vi "SwerveModuleOdometry.vi"(4 "Robot Heading(deg)":dbl, 6 "Wheel Distance (m)":dbl, 7 "Wheel Azimuth (deg)":dbl, 9 "Velocity (m/s)":dbl) -> (0 "Delta Y (m)":dbl, 1 "Delta X (m)":dbl, 2 "Velocity Y (m/s)":dbl, 3 "Velocity X (m/s)":dbl)   [LabVIEW 2020]
doc: "This VI calculates the odometry for a single swerve module."
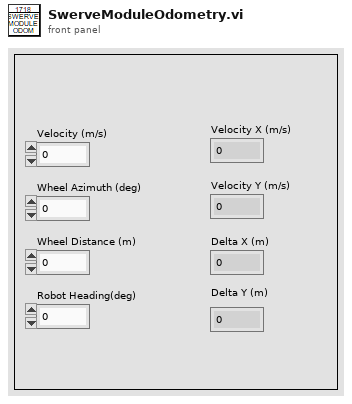
[diagram p1: front panel]
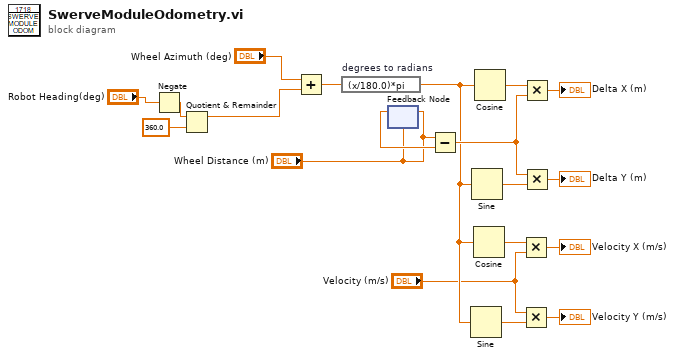
[diagram p0: block diagram]
diagram:
  n1 = Negate(x="Robot Heading(deg)") -> (-x=w1:dbl)
  n2 = Quotient & Remainder(x=w1, y=360.0) -> (x-y*floor(x/y)=w2:dbl)  [unwired: 1 out]
  n3 = Add(x="Wheel Azimuth (deg)", y=w2) -> (x+y=w15:dbl)
  n4 = expression code="(x/180.0)*pi" "degrees to radians"(w15) -> (w10:dbl)
  n5 = feedback #1("Wheel Distance (m)") -> (w14:dbl)
  n6 = feedback-in #1("Wheel Distance (m)") -> ()
  n7 = Subtract(x="Wheel Distance (m)", y=w14) -> (x-y=w17:dbl)
  n8 = Sine(x=w10) -> (sin(x)=w12:dbl)
  n9 = Sine(x=w10) -> (sin(x)=w18:dbl)
  n10 = Cosine(x=w10) -> (cos(x)=w11:dbl)
  n11 = Cosine(x=w10) -> (cos(x)=w16:dbl)
  n12 = Multiply(x=w11, y="Velocity (m/s)") -> (x*y=→"Velocity X (m/s)":dbl)
  n13 = Multiply(x="Velocity (m/s)", y=w12) -> (x*y=→"Velocity Y (m/s)":dbl)
  n14 = Multiply(x=w16, y=w17) -> (x*y=→"Delta X (m)":dbl)
  n15 = Multiply(x=w17, y=w18) -> (x*y=→"Delta Y (m)":dbl)
